vi "Google Map - Multiple String Locations Example.vi"() -> ()   [LabVIEW 2012]
uses:
  TypeDefs/Map Types.ctl
  TypeDefs/Marker Sizes.ctl
  TypeDefs/Marker Labels.ctl
panel:
  out "2D Picture":picture
  in  "System Stop Button":bool
  in  "Refresh":bool
  in  "Map Type":T1=enum."hybrid"
  in  "Color":u32(colorbox)=65793
  in  "Size":T2
  in  "Label":T3
  in  "Icon URL":string="http://lavag.org/public/style_extra/forum_imgs/LV.png"
  in  "Specify Icon?":bool=TRUE
  in  "Marker Location Array":string[](array[string])=["11500 N Mo-Pac Expy Austin, TX 78759", "32 Watershaugh Rd, Warkworth, Northumberland, England", "38 Penny Green St Sugar Land TX", "Rannes St, Insch, Scotland"]
  # "Marker Customization"
  # "or"
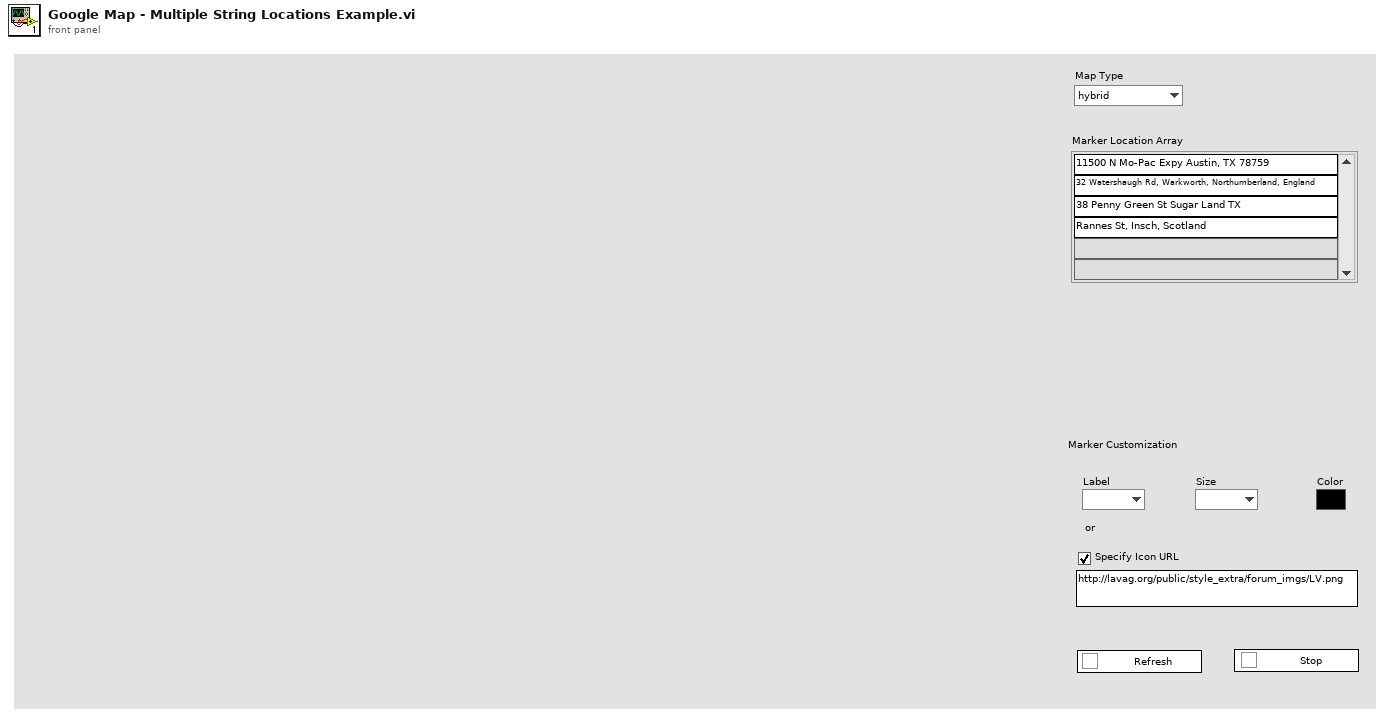
[diagram p1: front panel]
types:
  T1 = typedef "Map Types.ctl" = enum16{"roadmap", "satellite", "terrain", "hybrid"}
  T2 = typedef "Marker Sizes.ctl" = enum16{"", "small", "mid", "tiny"}
  T3 = typedef "Marker Labels.ctl" = enum16{"", "A", "B", "C", "D", "E", "F", "G", "H", "I", "J", "K", "M", "N", "O", "P", "Q", "R", "S", "T", "U", "V", "W", "X", "Y", "Z", "1", "2", "3", "4", "5", "6", "7", "8", "9", "0"}
  T4 = typedef "LVBoundsTypeDef.ctl" = cluster{"Width":u32, "Height":u32}
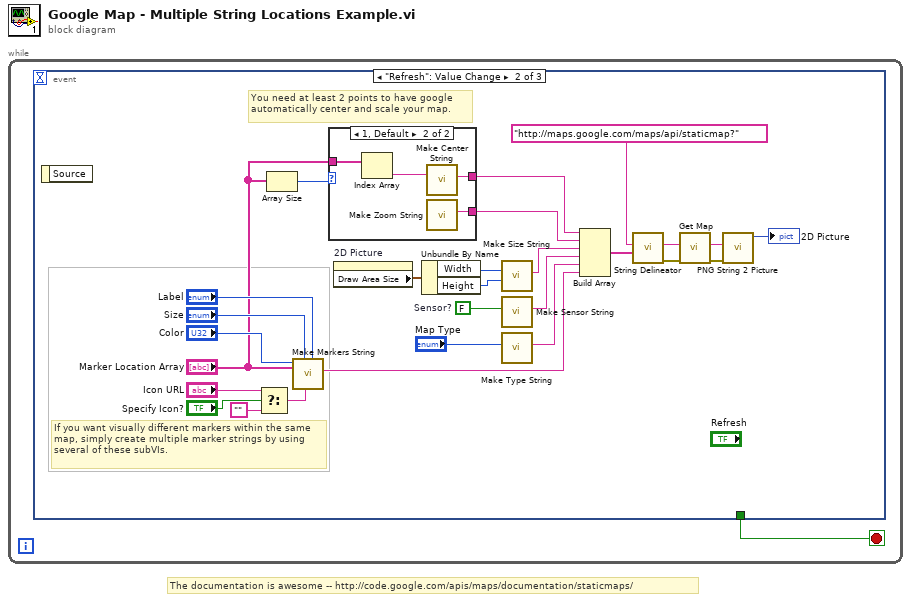
[diagram p0: block diagram]
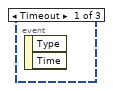
[diagram p2: hidden frame]
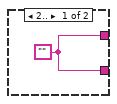
[diagram p3: hidden frame]
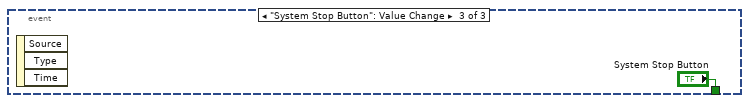
[diagram p4: hidden frame]
diagram:
  # "The documentation is awesome -- http://code.google.com/apis/maps/documentation/staticmaps/"
  n1 = while {
    stop <- w1 stop-if-true
    n2 = event shown="[1] \"Refresh\": Value Change" {
      selector: _ -> [_ _ _]
      dyn-events: _ -> [_ _ _]
      timeout: _ -> [_ _ _]
      tunnel: [_ _ "System Stop Button"] -> w1
      event Timeout {
        n3 = event-data() -> ()  [unwired: 1 in, 2 out]
      }
      event "Refresh": Value Change {
        w15 = FALSE  # Sensor?
        # "You need at least 2 points to have google automatically center and scale your map."
        # "If you want visually different markers within the same map, simply create multiple marker strings by using several of these subVIs."
        n4 = event-data() -> ()  [unwired: 1 in, 1 out]
        n5 = Select(t="Icon URL", s="Specify Icon?", f="") -> (s? t:f=w4:string)
        n6 = Array Size(array="Marker Location Array") -> (size(s)=w3:i32)
        n7 = call "Make Markers String.vi"("Label (optional)"="Label", "Icon URL (optional)"=w4, "Size (optional)"="Size", "Array of Locations"="Marker Location Array", "Color (optional)"="Color") -> ("Markers string"=w26:string)  [unwired: 5 in, 1 out]
        n8 = case shown="1, Default" w3 {
          tunnel: [w29 w33] -> w27
          tunnel: [w29 w32] -> w28
          tunnel: "Marker Location Array" -> [_ w31]
          frame 2.. {
            w29 = ""
          }
          frame 1, Default {
            n9 = Index Array(array=w31) -> (element=w30:string)  [unwired: 1 in]
            n10 = call "Make Center String.vi"("Location string"=w30) -> ("Center string"=w33:string)  [unwired: 9 in, 1 out]
            n11 = call "Make Zoom String.vi"() -> ("Zoom string"=w32:string)  [unwired: 10 in, 1 out]
          }
        }
        n12 = property on="2D Picture" class="Pict"() -> ("Draw Area Size"=w21:T4)  [unwired: 2 in, 2 out]
        n13 = Unbundle By Name(w21) -> ("Width"=w22:u32, "Height"=w23:u32)
        n14 = call "Make Size String.vi"("Height (480)"=w23, "Width (480)"=w22) -> ("Size string"=w16:string)  [unwired: 8 in, 1 out]
        n15 = call "Make Sensor String.vi"("Sensor?"=w15) -> ("Sensor string"=w17:string)  [unwired: 9 in, 1 out]
        n16 = call "Make Type String.vi"("Map Type"="Map Type") -> ("maptype string"=w19:string)  [unwired: 9 in, 1 out]
        n17 = Build Array(w27, w28, w16, w17, w19, w26) -> (w18:string[])
        n18 = call "String Delineator.vi"("Array of Strings"=w18, "Base String"="http://maps.google.com/maps/api/staticmap?" ("URL")) -> ("error in (no error)"=w24:errorcluster, "New String"=w25:string)  [unwired: 8 in]
        n19 = call "Get Map.vi"("error in (no error)"=w24, "URL"=w25) -> ("error out"=w13:errorcluster, "Body"=w12:string)  [unwired: 8 in]
        n20 = call "PNG String 2 Picture.vi"("error in (no error)"=w13, "PNG Data as String"=w12) -> ("Picture Out"=→"2D Picture":picture)  [unwired: 8 in, 1 out]
      }
      event "System Stop Button": Value Change {
        n21 = event-data() -> ()  [unwired: 1 in, 3 out]
      }
    }
  }
